vi "try_Sets and Maps.vi"() -> ()   [LabVIEW 2020]
panel:
  in  "Student Name":string
  in  "Student Name":string
  out "Age":i8
  out "Element in Map?":bool
  in  "Student Name":string
  in  "Delete":bool
  in  "Element in map?":bool
  in  "Age":i8
  in  "Insert Map":bool
  out "Set":set{dbl}(c389)
  in  "Stop":bool
  in  "Delete":dbl
  in  "Delete":bool
  out "Element in set?":bool
  in  "Element in set?":dbl
  in  "Element in set?":bool
  in  "Insert Set":dbl
  in  "Insert Set":bool
  out "Map (Students Age)":map{string, i32}(c390)
  # "Scenario\nSets and Maps are data types that allow for the storage of collections of data. Sets are ordered lists of the same data type, while Maps provide storage of key-value pairs with fast lookups.\n\nInstructions\n*For Set: Use the Insert control to insert an element, use the Is element in set? control to confirm if a number is within a set and use the Delete button to delete the element from the set\n*For Map: Use the Insert control to insert a Map entry with the Student Name and Age, use the Is element in map? control to confirm if a Student name is within the map and use the Delete button to delete the student entry from the map\n\n2. Run the VI"
  # "Set"
  # "Map"
  # "Insert Element"
  # "Insert Element"
  # "Find element"
  # "Find Student"
  # "Delete element"
  # "Delete element"
  # "Close this VI when you are done with the demo."
  # "You do not need to save changes to this VI."
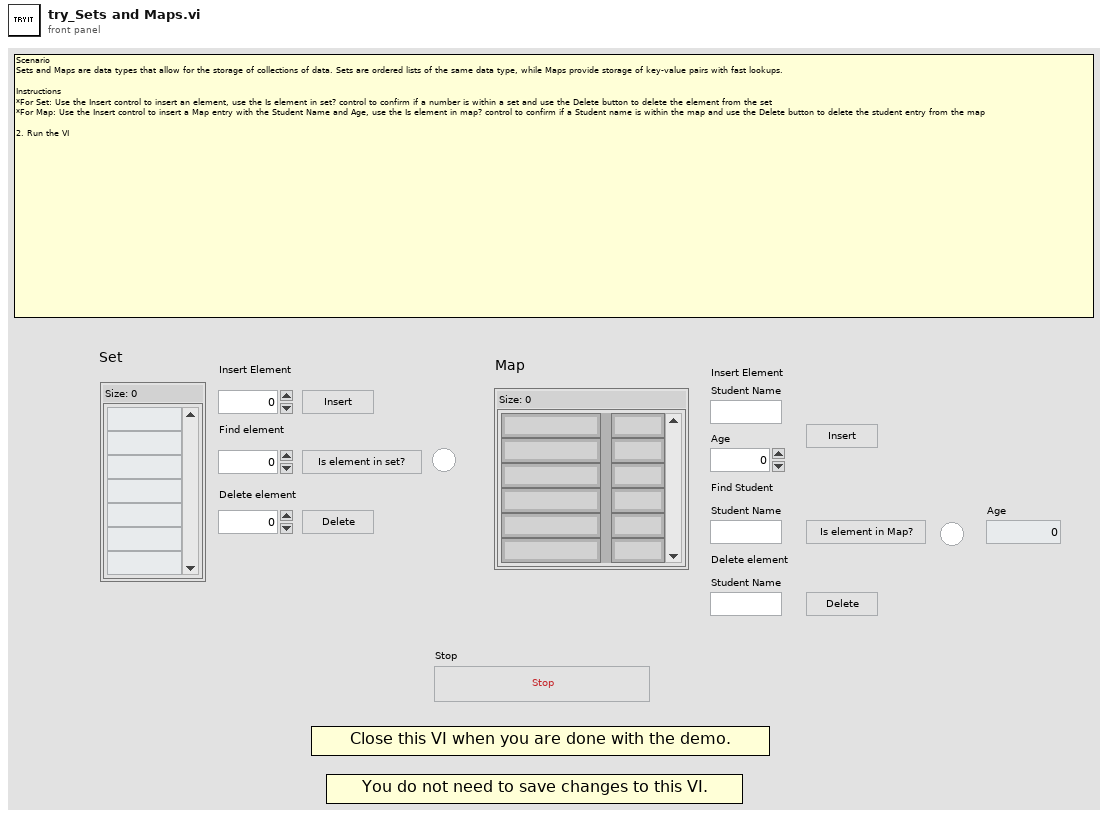
[diagram p1: front panel]
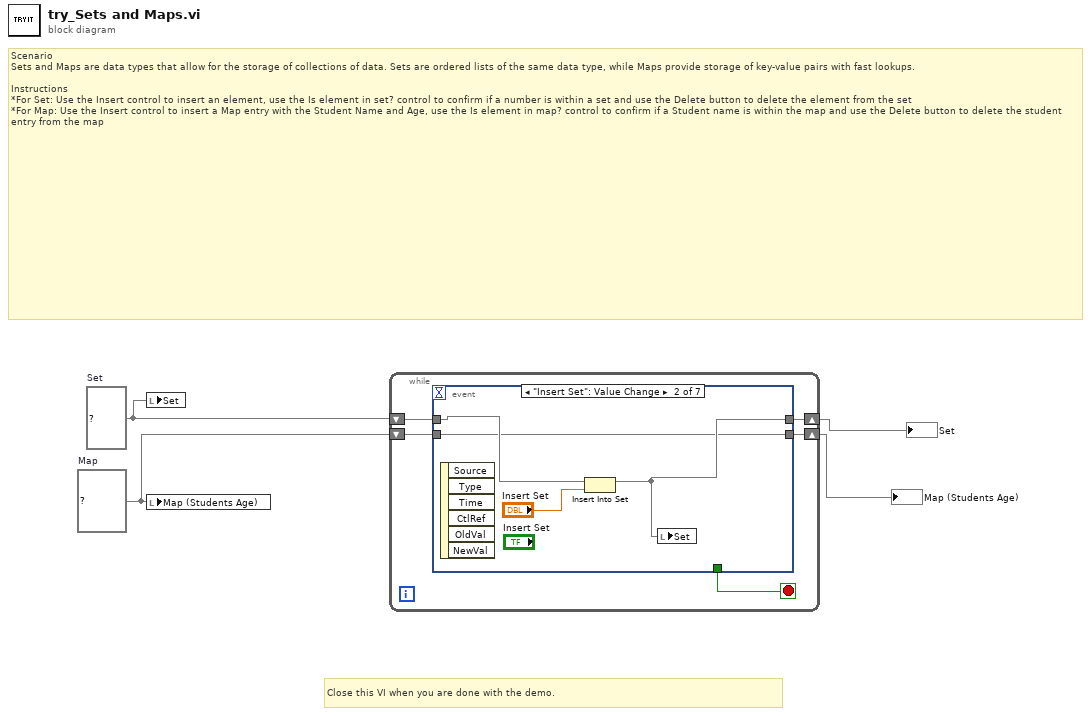
[diagram p0: block diagram]
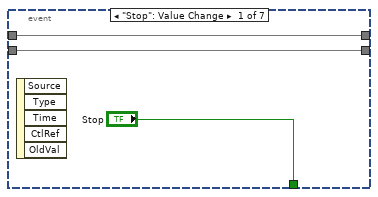
[diagram p2: hidden frame]
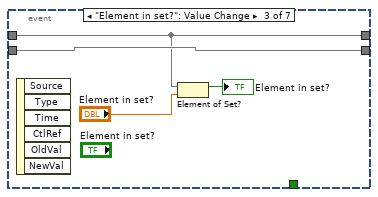
[diagram p3: hidden frame]
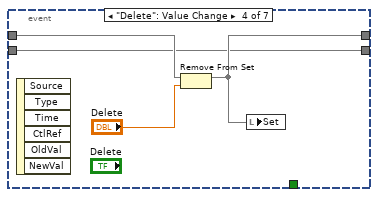
[diagram p4: hidden frame]
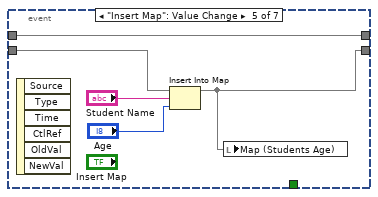
[diagram p5: hidden frame]
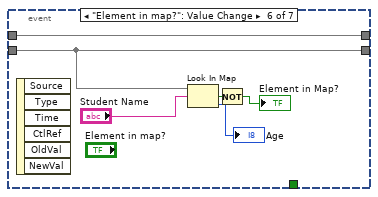
[diagram p6: hidden frame]
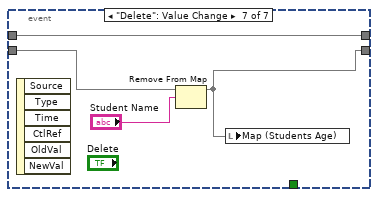
[diagram p7: hidden frame]
diagram:
  w4 = set{dbl} {}  # Set
  w3 = map{string, i32} {}  # Map
  # "Close this VI when you are done with the demo."
  # "Scenario\nSets and Maps are data types that allow for the storage of collections of data. Sets are ordered lists of the same data type, while Maps provide storage of key-value pairs with fast lookups.\n\nInstructions\n*For Set: Use the Insert control to insert an element, use the Is element in set? control to confirm if a number is within a set and use the Delete button to delete the element from the set\n*For Map: Use the Insert control to insert a Map entry with the Student Name and Age, use the Is element in map? control to confirm if a Student name is within the map and use the Delete button to delete the student entry from the map"
  n1 = local write "Set"(w4) -> ()
  n2 = local write "Map (Students Age)"(w3) -> ()
  n3 = while {
    shift-right: [w5] -> w1
    shift-left: w4 -> [w7]
    shift-right: [w8] -> w2
    shift-left: w3 -> [w6]
    stop <- w9 stop-if-true
    n4 = event shown="[1] \"Insert Set\": Value Change" {
      selector: _ -> [_ _ _ _ _ _ _]
      dyn-events: _ -> [_ _ _ _ _ _ _]
      timeout: _ -> [_ _ _ _ _ _ _]
      tunnel: ["Stop" _ _ _ _ _ _] -> w9
      tunnel: w6 -> [w11 w13 w20 w21 w26 w31 w37]
      tunnel: [w11 w13 w20 w21 w25 w31 w36] -> w8
      tunnel: w7 -> [w10 w15 w17 w23 w27 w30 w38]
      tunnel: [w10 w14 w17 w22 w27 w30 w38] -> w5
      event "Stop": Value Change {
        n5 = event-data() -> ()  [unwired: 1 in, 5 out]
      }
      event "Insert Set": Value Change {
        n6 = event-data() -> ()  [unwired: 1 in, 6 out]
        n7 = Insert Into Set(10:"Insert Set", 11:w15) -> (3:w14:set{dbl})  [unwired: 1 out]
        n8 = local write "Set"(w14) -> ()
      }
      event "Element in set?": Value Change {
        n9 = event-data() -> ()  [unwired: 1 in, 6 out]
        n10 = Element of Set?(10:"Element in set?", 11:w17) -> (3:→"Element in set?":bool)
      }
      event "Delete": Value Change {
        n11 = event-data() -> ()  [unwired: 1 in, 6 out]
        n12 = Remove From Set(10:"Delete", 11:w23) -> (3:w22:set{dbl})  [unwired: 1 out]
        n13 = local write "Set"(w22) -> ()
      }
      event "Insert Map": Value Change {
        n14 = event-data() -> ()  [unwired: 1 in, 6 out]
        n15 = Insert Into Map(map in=w26, key="Student Name", value="Age") -> (map out=w25:map{string, i32})  [unwired: 2 out]
        n16 = local write "Map (Students Age)"(w25) -> ()
      }
      event "Element in map?": Value Change {
        n17 = event-data() -> ()  [unwired: 1 in, 6 out]
        n18 = Look In Map(map=w31, key="Student Name") -> (key not found?=w33:bool, value=→"Age":i32)  [unwired: 1 in]
        n19 = Not(x=w33) -> (.not. x?=→"Element in Map?":bool)
      }
      event "Delete": Value Change {
        n20 = event-data() -> ()  [unwired: 1 in, 6 out]
        n21 = Remove From Map(10:"Student Name", 11:w37) -> (3:w36:map{string, i32})  [unwired: 2 out]
        n22 = local write "Map (Students Age)"(w36) -> ()
      }
    }
  }
  "Map (Students Age)" <- w2
  "Set" <- w1
